vi "Server Routing Loop.vi"(8 "error in (no error)":errorcluster, 11 "TCPMessaging in":refnum<class "TCPMessaging.lvclass">) -> (0 "error out":errorcluster)   [LabVIEW 2020, in "Vecto.lvlib" / "TCPMessaging.lvclass"]
doc: "Routes outgoing payloads to the correct client."
uses:
  TCPMessaging.lvclass
  TCPMessaging.lvclass/TCPMessaging.ctl
  SequenceCountService/SequenceCountService.lvclass
  Vecto.lvlib
  proto/TcpPayload/TcpPayload.lvlib
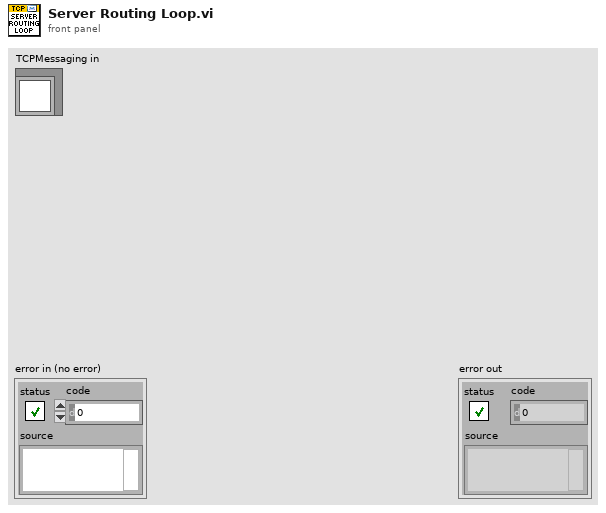
[diagram p1: front panel]
types:
  T1 = typedef "Vecto.lvlib/TX Payload.ctl" = cluster{"Target ID":u32, "Payload":string}
  T2 = typedef "Vecto.lvlib/Send Message Data.ctl" = cluster{"TcpPayload":T3, "Register Reply":bool, "Reply Promise":refnum<class "Promise.lvclass">, "Reply Deadline":dbl}
  T3 = typedef "TcpPayload.lvlib/Data.ctl" = cluster{"target_node":u32, "target_task":u32, "source_id":u32, "sequence":u32, "timestamp":u64, "type_id":u32, "payload":u8[]}
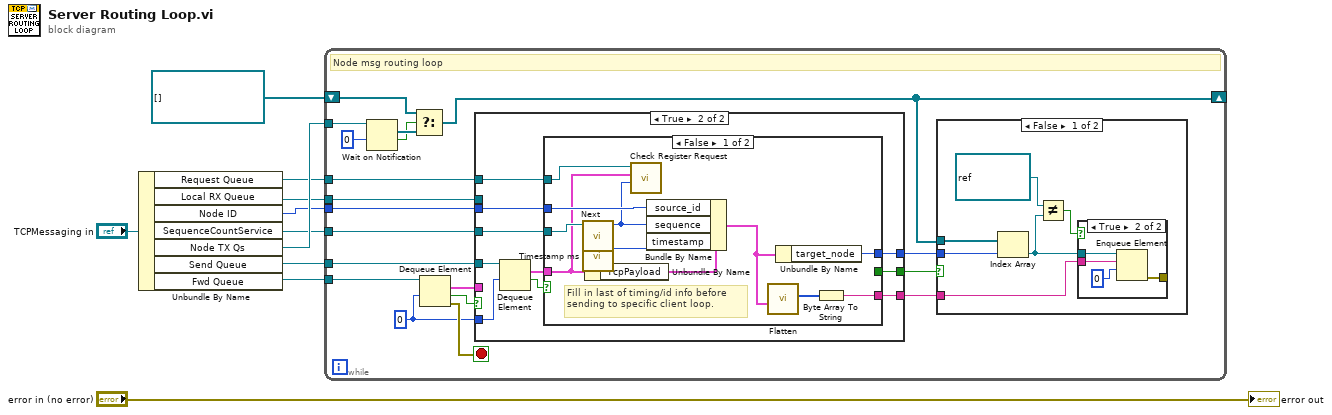
[diagram p0: block diagram]
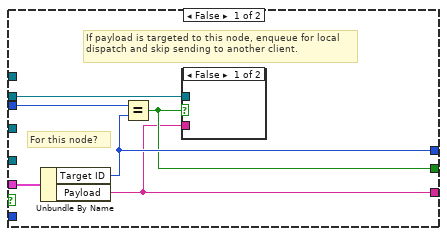
[diagram p4: hidden frame]
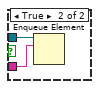
[diagram p5: hidden frame]
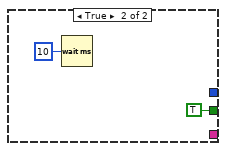
[diagram p6: hidden frame]
diagram:
  n1 = Unbundle By Name("TCPMessaging in") -> ("Request Queue"=w1:refnum<queue>, "Local RX Queue"=w2:refnum<queue>, "Node ID"=w4:u32, "SequenceCountService"=w3:refnum<class "SequenceCountService.lvclass">, "Node TX Qs"=w7:refnum<notifier>, "Send Queue"=w8:refnum<queue>, "Fwd Queue"=w5:refnum<queue>)
  n2 = while {
    tunnel: w8 -> [w28]
    tunnel: w7 -> [w27]
    shift-right: [w14] -> _
    shift-left: refnum<queue>[] [] ("queue out") -> [w23]
    tunnel: w5 -> [w22]
    tunnel: w4 -> [w17]
    tunnel: w3 -> [w16]
    tunnel: w2 -> [w12]
    tunnel: w1 -> [w11]
    stop <- w29 stop-if-true
    w21 = 0 ("timeout in ms (-1)")
    # "Node msg routing loop"
    n3 = Wait on Notification(notifier=w27, timeout in ms (-1)=0) -> (notification=w25:refnum<queue>[], timed out?=w24:bool)  [unwired: 2 in, 2 out]
    n4 = Select(t=w23, s=w24, f=w25) -> (s? t:f=w14:refnum<queue>[])
    n5 = Dequeue Element(queue=w22, timeout in ms (-1)=w21) -> (element=w19:T1, timed out?=w20:bool, error out=w29:errorcluster)  [unwired: 1 in, 1 out]
    n6 = case shown="True" w20 {
      tunnel: w28 -> [_ w57]
      tunnel: w21 -> [_ w55]
      tunnel: w19 -> [w45 _]
      tunnel: [w44 w50] -> w18
      tunnel: w17 -> [w43 w53]
      tunnel: w16 -> [_ w52]
      tunnel: [w40 w51] -> w15
      tunnel: [w41 w49] -> w13
      tunnel: w12 -> [w42 _]
      tunnel: w11 -> [_ w48]
      frame False {
        # "If payload is targeted to this node, enqueue for local dispatch and skip sending to another client."
        # "For this node?"
        n7 = Unbundle By Name(w45) -> ("Target ID"=w44:u32, "Payload"=w40:string)
        n8 = Equal?(x=w43, y=w44) -> (x = y?=w41:bool)
        n9 = case shown="False" w41 {
          tunnel: w42 -> [_ w47]
          tunnel: w40 -> [_ w46]
          frame False {
          }
          frame True {
            n10 = Enqueue Element(queue=w47, element=w46) -> ()  [unwired: 2 in, 3 out]
          }
        }
      }
      frame True {
        n11 = Dequeue Element(queue=w57, timeout in ms (-1)=w55) -> (element=w56:T2, timed out?=w54:bool)  [unwired: 1 in, 2 out]
        n12 = case shown="False" w54 {
          tunnel: w56 -> [w59 _]
          tunnel: w53 -> [w68 _]
          tunnel: w52 -> [w67 _]
          tunnel: [w65 _] -> w51
          tunnel: [w62 _] -> w50
          tunnel: [_ TRUE] -> w49
          tunnel: w48 -> [w58 _]
          frame False {
            # "Fill in last of timing/id info before sending to specific client loop."
            n13 = call "Next.vi"("SequenceCountService in"=w67) -> ("Sequence"=w60:u32)  [unwired: 9 in, 1 out]
            n14 = call "Timestamp ms.vi"() -> ("Timestamp ms"=w66:u64)  [unwired: 7 in]
            n15 = Unbundle By Name(w59) -> ("TcpPayload"=w61:T3)
            n16 = call "Check Register Request.vi"("Sequence"=w60, "Send Message Data"=w59, "Request Queue"=w58) -> ()  [unwired: 8 in, 1 out]
            n17 = Bundle By Name(cluster=w61, "source_id"=w68, "sequence"=w60, "timestamp"=w66) -> (w63:T3)
            n18 = call "Flatten.vi"("Data"=w63) -> ("Buffer"=w64:u8[])  [unwired: 9 in, 1 out]
            n19 = Unbundle By Name(w63) -> ("target_node"=w62:u32)
            n20 = Byte Array To String(unsigned byte array=w64) -> (string=w65:string)
          }
          frame True {
            n21 = Wait (ms)(milliseconds to wait=u32 10) -> ()  [unwired: 1 out]
          }
        }
      }
    }
    n22 = case shown="False" w13 {
      tunnel: w18 -> [w33 _]
      tunnel: w15 -> [w32 _]
      tunnel: w14 -> [w30 _]
      frame False {
        n23 = Index Array(array=w30, index=w33) -> (element=w35:refnum<queue>)
        n24 = Not Equal?(x=refnum<queue> refnum ("queue out"), y=w35) -> (x != y?=w31:bool)
        n25 = case shown="True" w31 {
          tunnel: w32 -> [_ w39]
          tunnel: w35 -> [_ w38]
          tunnel: [_ w36] -> _
          frame False {
          }
          frame True {
            n26 = Enqueue Element(queue=w38, element=w39, timeout in ms (-1)=0) -> (error out=w36:errorcluster)  [unwired: 1 in, 2 out]
          }
        }
      }
      frame True {
        # "Sending message is skipped"
      }
    }
  }
  "error out" <- "error in (no error)"
